vi "VA CoAP - Message - Option Insert - 3 Uri-Host.vi"(7 "CoAP Server Address":string, 9 "Current Option Delta":u8, 10 "CoAP Message IN":string) -> (2 "New Option Delta":u8, 3 "CoAP Message OUT":string)   [LabVIEW 2020]
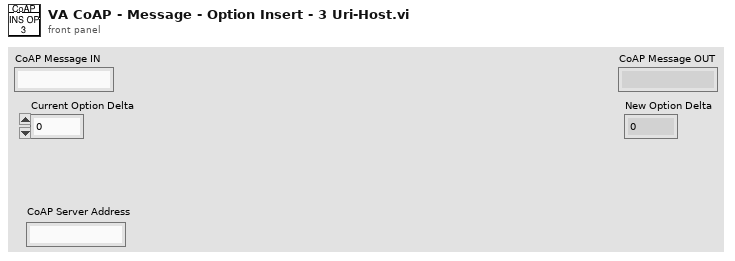
[diagram p1: front panel]
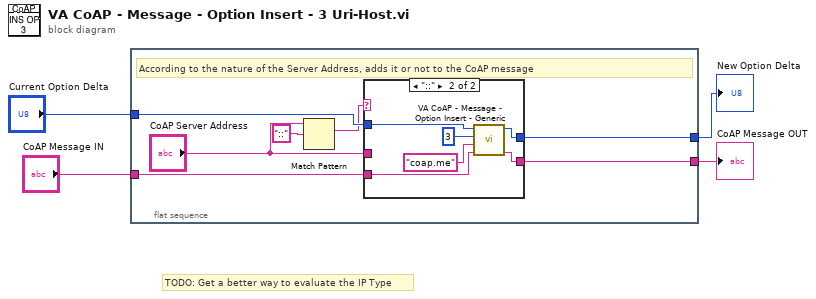
[diagram p0: block diagram]
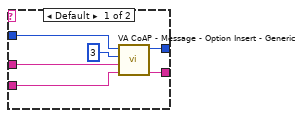
[diagram p2: hidden frame]
diagram:
  # "TODO: Get a better way to evaluate the IP Type"
  n1 = flat-sequence {
    tunnel: "CoAP Message IN" -> [w11]
    tunnel: [w10] -> w3
    tunnel: "Current Option Delta" -> [w9]
    tunnel: [w8] -> w1
    frame #0 {
      # "According to the nature of the Server Address, adds it or not to the CoAP message"
      n2 = Match Pattern(string="CoAP Server Address", regular expression="::") -> (match substring=w5:string)  [unwired: 1 in, 3 out]
      n3 = case shown="\"::\"" w5 {
        tunnel: w11 -> [w13 w19]
        tunnel: [w14 w20] -> w10
        tunnel: w9 -> [w15 w21]
        tunnel: [w16 w22] -> w8
        tunnel: "CoAP Server Address" -> [w12 _]
        frame Default {
          n4 = call "VA CoAP - Message - Option Insert - Generic.vi"("CoAP Message IN"=w13, "New Message Element"=w12, "Current Delta on Evaluation"=u8 3 ("Current Option Delta"), "Current Option Delta in"=w15) -> ("CoAP Message OUT"=w14:string, "Current Option Delta out"=w16:u8)  [unwired: 6 in]
        }
        frame "::" {
          n5 = call "VA CoAP - Message - Option Insert - Generic.vi"("CoAP Message IN"=w19, "New Message Element"="coap.me", "Current Delta on Evaluation"=u8 3 ("Current Option Delta"), "Current Option Delta in"=w21) -> ("CoAP Message OUT"=w20:string, "Current Option Delta out"=w22:u8)  [unwired: 6 in]
        }
      }
    }
  }
  "CoAP Message OUT" <- w3
  "New Option Delta" <- w1
